vi "FFT_Xilinx.vi"(11 "Inputs":T2) -> (3 "Outputs":T1)   [LabVIEW 2018]
uses:
  <vilib>/rvi/XilinxIP/XIPIN_XNode/niFpgaXIPIN.xnode
  FFT_Xilinx/FFT_1_0_0/xsim.dir/FFT_1_0_0_8C0FCDCCE72D4EB5AC3BB88B1A18D427/xsimk_8C0FCDCCE72D4EB5AC3BB88B1A18D427.dll
  <vilib>/rvi/IPIntegrationNode/IPINode_Xnode/niFpgaIPINode.xnode
  <vilib>/rvi/IPIntegrationNode/IPINode_Typedef/niFpgaIPINodeSupportedFamilies.ctl
  <vilib>/rvi/IPIntegrationNode/IPINode_Utilities/niFpgaIPINodeSimCore.vi
  FFT_Xilinx/FFT_Outputs.ctl
  FFT_Xilinx/FFT_Inputs.ctl
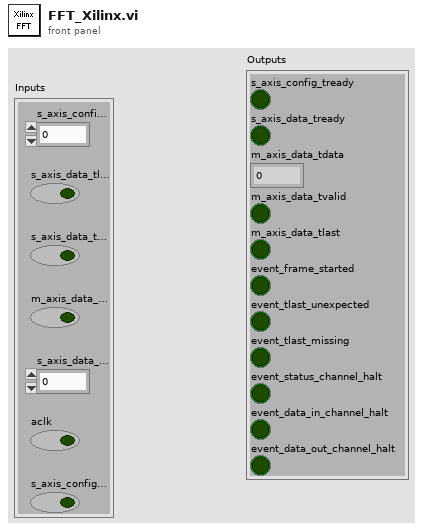
[diagram p1: front panel]
types:
  T1 = typedef "FFT_Outputs.ctl" = cluster{"s_axis_config_tready":bool, "s_axis_data_tready":bool, "m_axis_data_tdata":fxp<+,32,2>, "m_axis_data_tvalid":bool, "m_axis_data_tlast":bool, "event_frame_started":bool, "event_tlast_unexpected":bool, "event_tlast_missing":bool, "event_status_channel_halt":bool, "event_data_in_channel_halt":bool, "event_data_out_channel_halt":bool}
  T2 = typedef "FFT_Inputs.ctl" = cluster{"s_axis_config_tdata":fxp<+/-,16,1>, "s_axis_data_tdata":fxp<+/-,32,1>, "s_axis_data_tvalid":bool, "aclk":bool, "s_axis_config_tvalid":bool, "s_axis_data_tlast":bool, "m_axis_data_tready":bool}
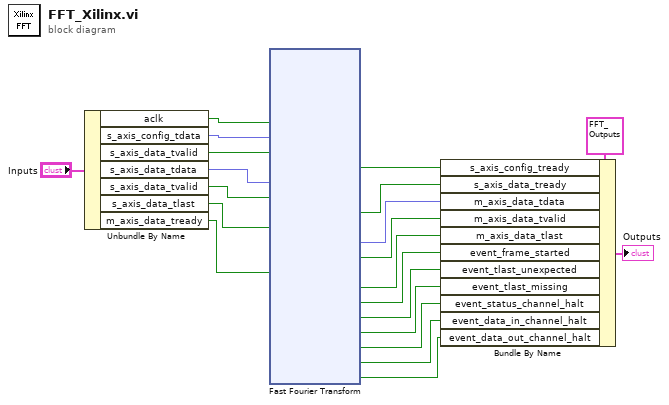
[diagram p0: block diagram]
diagram:
  n1 = Unbundle By Name("Inputs") -> ("aclk"=w20:bool, "s_axis_config_tdata"=w19:fxp<+/-,16,1>, "s_axis_data_tvalid"=w18:bool, "s_axis_data_tdata"=w17:fxp<+/-,32,1>, "s_axis_data_tvalid"=w16:bool, "s_axis_data_tlast"=w15:bool, "m_axis_data_tready"=w14:bool)
  n2 = xnode ("Fast Fourier Transform")("aclk"=w20, "s_axis_config_tdata"=w19, "s_axis_config_tvalid"=w18, "s_axis_data_tdata"=w17, "s_axis_data_tvalid"=w16, "s_axis_data_tlast"=w15, "m_axis_data_tready"=w14) -> ("s_axis_config_tready"=w11:bool, "s_axis_data_tready"=w10:bool, "m_axis_data_tdata"=w9:fxp<+,32,2>, "m_axis_data_tvalid"=w8:bool, "m_axis_data_tlast"=w7:bool, "event_frame_started"=w6:bool, "event_tlast_unexpected"=w5:bool, "event_tlast_missing"=w4:bool, "event_status_channel_halt"=w3:bool, "event_data_in_channel_halt"=w2:bool, "event_data_out_channel_halt"=w1:bool)
  n3 = Bundle By Name(cluster=T1 {"s_axis_config_tready"=FALSE, "s_axis_data_tready"=FALSE, "m_axis_data_tdata"=0.0, "m_axis_data_tvalid"=FALSE, "m_axis_data_tlast"=FALSE, "event_frame_started"=FALSE, "event_tlast_unexpected"=FALSE, "event_tlast_missing"=FALSE, "event_status_channel_halt"=FALSE, "event_data_in_channel_halt"=FALSE, "event_data_out_channel_halt"=FALSE} ("Cluster 2"), "s_axis_config_tready"=w11, "s_axis_data_tready"=w10, "m_axis_data_tdata"=w9, "m_axis_data_tvalid"=w8, "m_axis_data_tlast"=w7, "event_frame_started"=w6, "event_tlast_unexpected"=w5, "event_tlast_missing"=w4, "event_status_channel_halt"=w3, "event_data_in_channel_halt"=w2, "event_data_out_channel_halt"=w1) -> (→"Outputs":T1)
